vi "NChannelRunningAverage.vi"() -> ()   [LabVIEW 2012]
panel:
  in  "N point average":i32=20 min=0
  out "Waveform Chart":dbl[][](graph)
  in  "stop":bool
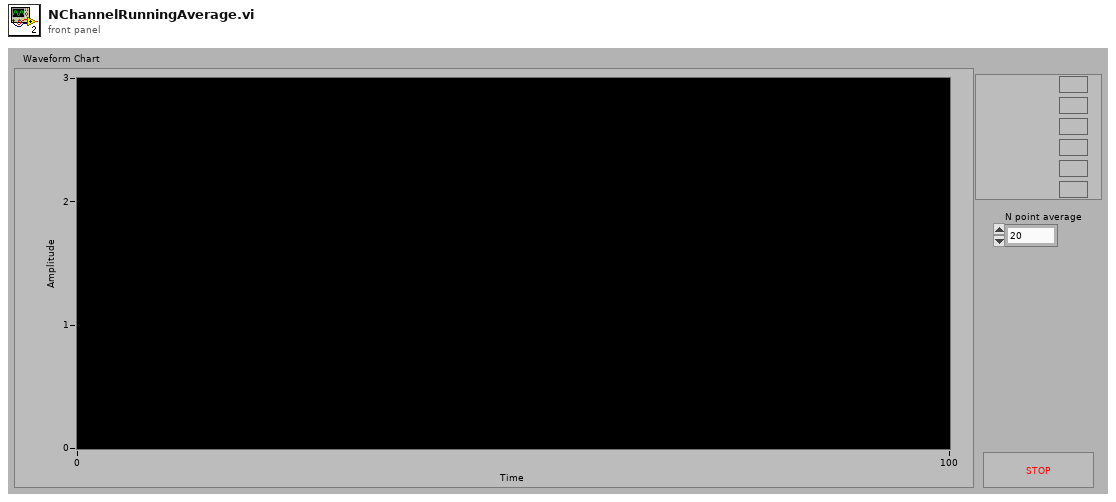
[diagram p1: front panel]
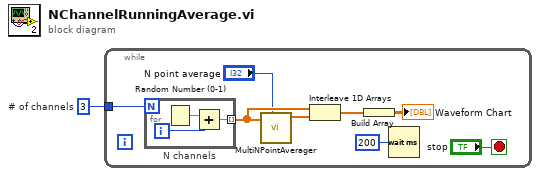
[diagram p0: block diagram]
diagram:
  w1 = 3  # # of channels
  n1 = while {
    tunnel: w1 -> [w7]
    stop <- "stop" stop-if-true
    n2 = for "N channels" {
      N: w7 -> [_]
      tunnel: [w11] -> w3 mode=indexing
      i -> [w10]
      n3 = Random Number (0-1) ("New data")() -> (number: 0 to 1=w12:dbl)
      n4 = Add(x=w12, y=w10) -> (x+y=w11:dbl)
    }
    n5 = call "MultiNPointAverager.vi"("N point average"="N point average", "Array of values"=w3) -> ("Array of averages"=w5:dbl[])  [unwired: 9 in]
    n6 = Interleave 1D Arrays(w3, w5) -> (w4:dbl[])
    n7 = Build Array(w4) -> (→"Waveform Chart":dbl[][])
    n8 = Wait (ms)(milliseconds to wait=u32 200) -> ()  [unwired: 1 out]
  }
